vi "UART.vi"() -> ()   [LabVIEW 2020]
uses:
  <vilib>/Instr/_visa.llb/VISA Configure Serial Port (Instr).vi
panel:
  in  "stop":bool
  out "String 2":string
  in  "VISA resource name":refnum<visa-resource-name>
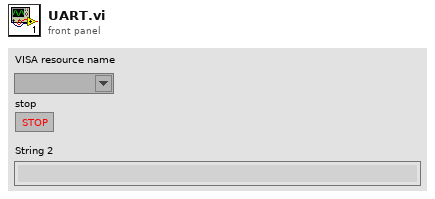
[diagram p1: front panel]
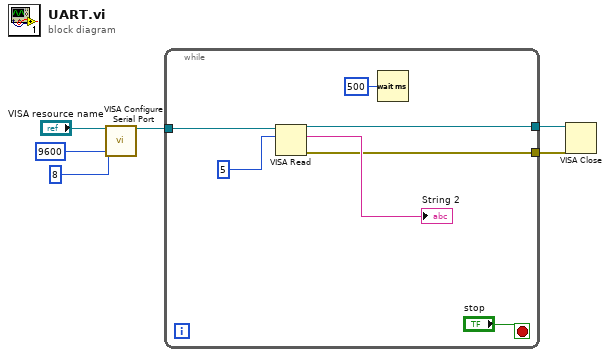
[diagram p0: block diagram]
diagram:
  n1 = call-poly "VISA Configure Serial Port"("VISA resource name"="VISA resource name", "baud rate (9600)"=u32 9600, "data bits (8)"=u16 8) -> ("VISA resource name out"=w3:refnum<visa-resource-name>)  [unwired: 11 in, 1 out]
  n2 = while {
    tunnel: w3 -> [w13]
    tunnel: [w9] -> w2
    tunnel: [w7] -> w1
    stop <- "stop" stop-if-true
    n3 = VISA Read(VISA resource name=w13, byte count=u32 5) -> (VISA resource name out=w9:refnum<visa-resource-name>, read buffer=→"String 2":string, error out=w7:errorcluster)  [unwired: 1 in, 1 out]
    n4 = Wait (ms)(milliseconds to wait=u32 500) -> ()  [unwired: 1 out]
  }
  n5 = VISA Close(VISA resource name=w2, error in (no error)=w1) -> ()  [unwired: 1 out]
